vi "EIS_Create.vi"(0 "reference in":refnum<class "EIS.lvclass">, 5 "EIS Parameters":T1={"EIS Mode"=2, "EIS DC Potential"=650.0, "EIS Start Frequency"=1000.0, "EIS Stop Frequency"=500.0, "EIS Delta Frequency"=100.0, "EIS DC Current"=0.0, "AC Signal (mV/mA RMS)"=20.0, "Cycles at Frequency"=1000.0, "EIS AC Step Delay"=1.0} {"EIS Mode" items=["Voltage (PEIS)"=1, "Current (GEIS)"=2]}, 7 "Logger":refnum<class "Logger.lvclass">, 9 "HPS17K Refs":refnum<class "HPS-17000.lvclass">[](array[class]), 11 "Error In":errorcluster) -> (4 "reference out":refnum<class "EIS.lvclass">, 6 "ProcessViRef":refnum<vi>, 15 "Error Out":errorcluster)   [LabVIEW 2023, in "EIS.lvclass"]
uses:
  EIS.lvclass
  Types/EIS Parameters.ctl
  Types/EIS Mode.ctl
  Logger_class/Logger.lvclass
  <instrlib>/HPS-17000/HPS-17000.lvclass
  EIS.lvclass/EIS.ctl
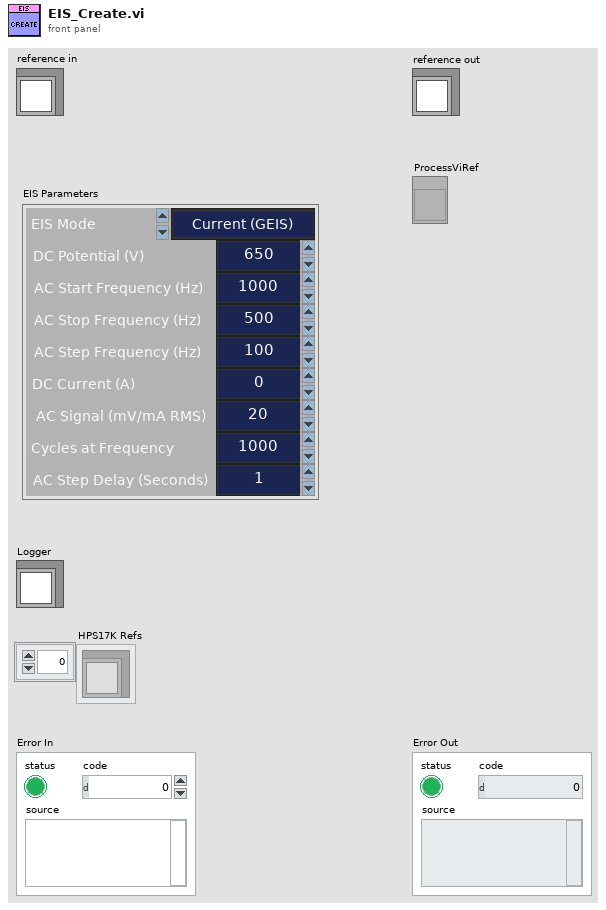
[diagram p1: front panel]
types:
  T1 = typedef "EIS Parameters.ctl" = cluster{"EIS Mode":T2, "EIS DC Potential":dbl, "EIS Start Frequency":dbl, "EIS Stop Frequency":dbl, "EIS Delta Frequency":dbl, "EIS DC Current":dbl, "AC Signal (mV/mA RMS)":dbl, "Cycles at Frequency":dbl, "EIS AC Step Delay":dbl}
  T2 = typedef "EIS Mode.ctl" = u16
  T3 = typedef "EIS.lvclass/ObjectAttributes.ctl" = cluster{"EIS Parameters":T1, "Logger":refnum<class "Logger.lvclass">, "HPS17K Refs":refnum<class "HPS-17000.lvclass">[]}
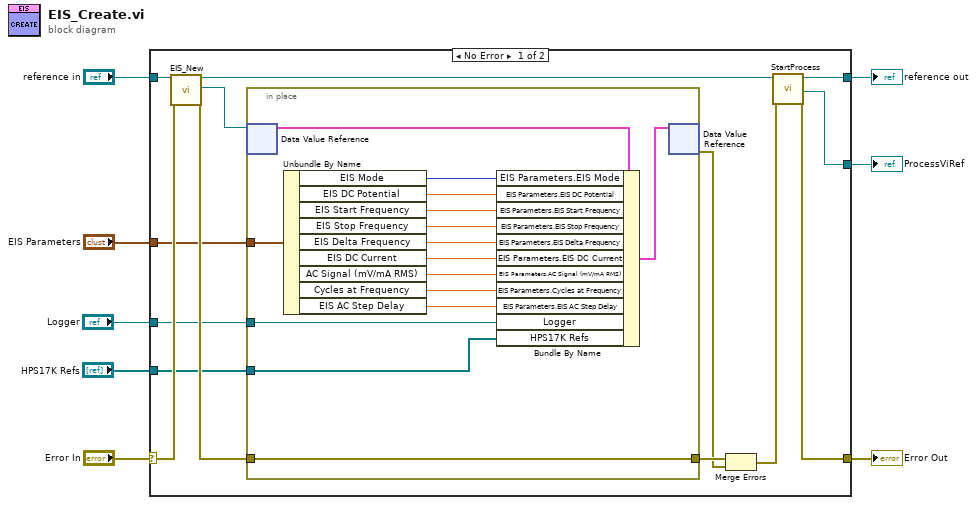
[diagram p0: block diagram]
diagram:
  n1 = case shown="No Error" "Error In" {
    selector: "Error In" -> [w21 w39]
    tunnel: [w15 w39] -> w7
    tunnel: "reference in" -> [w22 w38]
    tunnel: [w17 w38] -> w5
    tunnel: [w14 _] -> w4
    tunnel: "EIS Parameters" -> [w13 _]
    tunnel: "Logger" -> [w10 _]
    tunnel: "HPS17K Refs" -> [w9 _]
    frame No Error {
      n2 = call "EIS_New.vi"("reference in"=w22, "Error In"=w21) -> ("reference out"=w18:refnum<class "EIS.lvclass">, "DVRRefOut"=w12:refnum<data-value>, "Error Out"=w20:errorcluster)  [unwired: 14 in, 1 out]
      n3 = in-place {
        in-place-border: w20 -> [w37]
        in-place-border: [w37] -> w19
        in-place-border: w13 -> [w34]
        in-place-border: w10 -> [w24]
        in-place-border: w9 -> [w23]
        n4 = in-place-dvr #1(w12) -> (w36:T3)  [unwired: 1 out]
        n5 = Unbundle By Name(w34) -> ("EIS Mode"=w33:T2, "EIS DC Potential"=w32:dbl, "EIS Start Frequency"=w31:dbl, "EIS Stop Frequency"=w30:dbl, "EIS Delta Frequency"=w29:dbl, "EIS DC Current"=w28:dbl, "AC Signal (mV/mA RMS)"=w27:dbl, "Cycles at Frequency"=w26:dbl, "EIS AC Step Delay"=w25:dbl)
        n6 = Bundle By Name(cluster=w36, "EIS Parameters.EIS Mode"=w33, "EIS Parameters.EIS DC Potential"=w32, "EIS Parameters.EIS Start Frequency"=w31, "EIS Parameters.EIS Stop Frequency"=w30, "EIS Parameters.EIS Delta Frequency"=w29, "EIS Parameters.EIS DC Current"=w28, "EIS Parameters.AC Signal (mV/mA RMS)"=w27, "EIS Parameters.Cycles at Frequency"=w26, "EIS Parameters.EIS AC Step Delay"=w25, "Logger"=w24, "HPS17K Refs"=w23) -> (w35:T3)
        n7 = in-place-dvr #1(w35) -> (w11:errorcluster)  [unwired: 1 out]
      }
      n8 = Merge Errors(w19, w11) -> (w16:errorcluster)
      n9 = call "StartProcess.vi"("reference in"=w18, "Error In"=w16) -> ("reference out"=w17:refnum<class "EIS.lvclass">, "ProcessViRef"=w14:refnum<vi>, "Error Out"=w15:errorcluster)  [unwired: 13 in, 2 out]
    }
    frame Error {
      # "VI-TechBaseTemplate_Simple_6x8x6"
    }
  }
  "Error Out" <- w7
  "reference out" <- w5
  "ProcessViRef" <- w4
